vi "Bool String.vi"(4 "Bool":bool) -> (7 "String":string)   [LabVIEW 2024, in "CTI.lvlib" / "VisaComms.lvclass"]
uses:
  VisaComms.lvclass
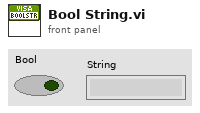
[diagram p1: front panel]
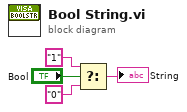
[diagram p0: block diagram]
diagram:
  n1 = Select(t="1", s="Bool", f="0") -> (s? t:f=→"String":string)
